vi "GPSDO53335ATester.vi"() -> ()   [LabVIEW 2015]
uses:
  <vilib>/Instr/_visa.llb/VISA Configure Serial Port (Instr).vi
panel:
  out "Measurement":cluster{"Measurment":ext, "Measurment":ext}(graph)
  out "Measurment":ext format="%.9e"
  in  "AC\nDC 2":bool
  in  "AC\nDC":bool
  in  "Gate Delay":ext=0.25 format="%.3f"
  out "CNT No Change Votes":dbl
  out "CNT Down Votes":dbl
  out "CNT Up Votes":dbl
  out "RS No Change Votes":dbl
  out "RS Down Votes":dbl
  out "Running Sum":dbl(graph)
  in  "Clear":bool
  in  "Baud Rate":dbl=115200.0
  in  "COM Port":refnum<visa-resource-name>
  out "Error Out":errorcluster
  in  "Error In":errorcluster
  out "Tracked Satellites":cluster{dbl, dbl}(graph)
  in  "Save DAC to EEPROM":bool
  in  "Reset GPS":bool
  in  "Set DAC":dbl
  in  "Update DAC":bool
  in  "Change Algorithim":bool
  out "UpTime":string
  out "Warmed Up?":bool
  out "Enforce Warmup":bool
  out "Algorithim In Use":string
  out "Antenna Status":string
  out "Time":string
  in  "Stop":bool
  out "Raw Data":string
  out "Date":string
  out "RS Up Votes":dbl
  out "Running Sum":dbl
  out "DAC Value":dbl
  out "Adjustments Made":dbl
  out "Samples":dbl
  out "Error (mHz)":dbl
  out "Count":cluster{dbl, dbl}(graph)
  out "Longitude":dbl format="%#_9g"
  out "Latitude":dbl
  out "Tracked Satellites":dbl
  out "Visible Satellites":dbl
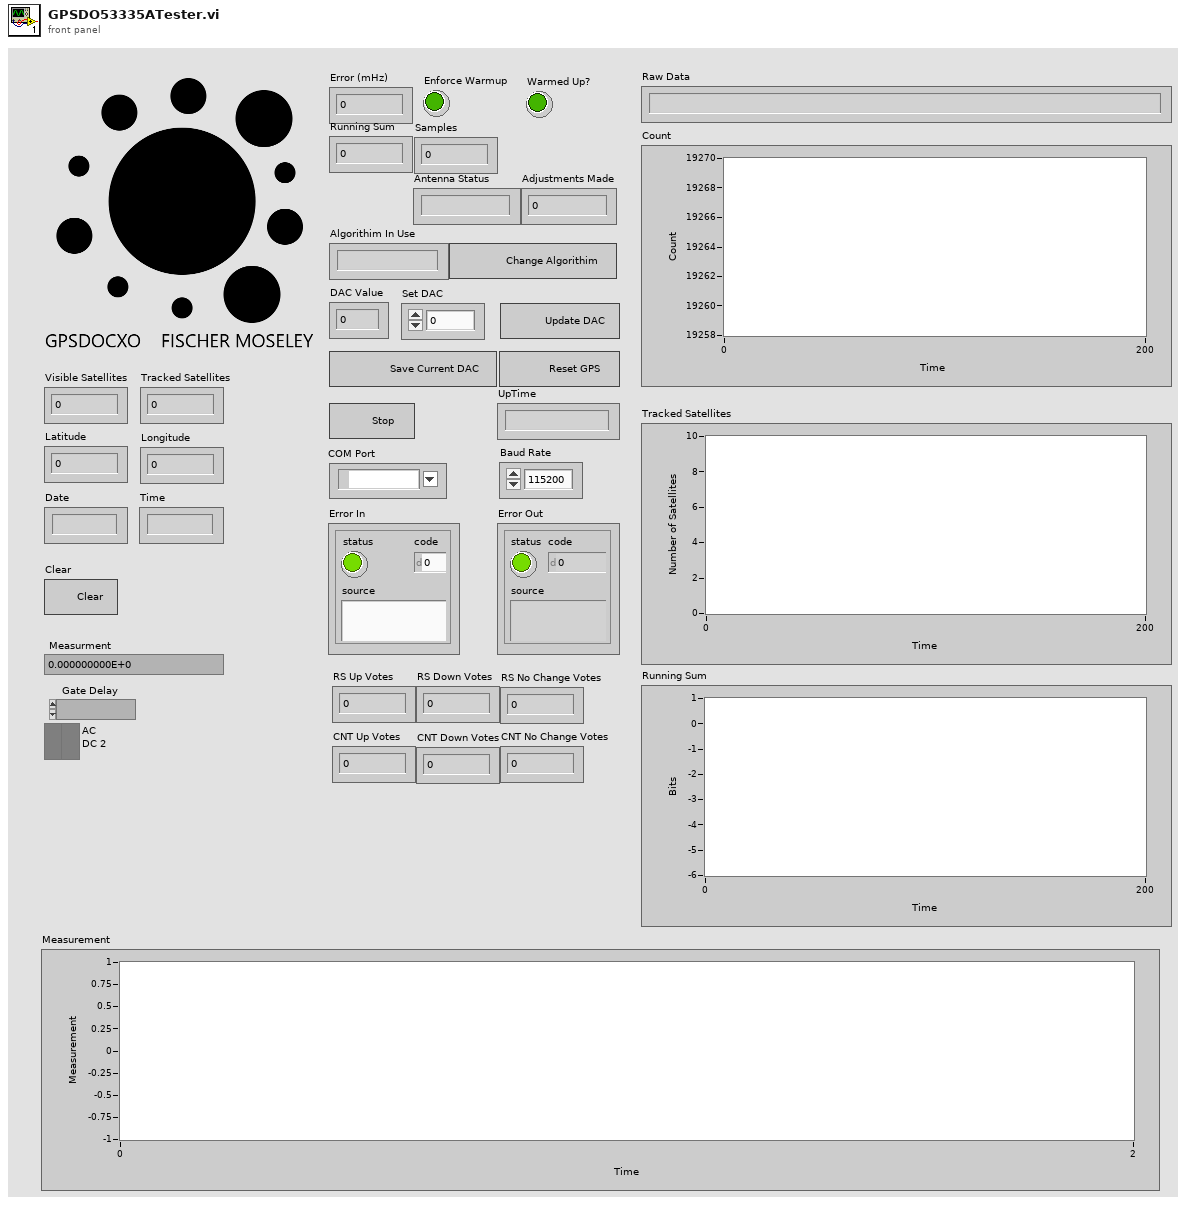
[diagram p1: front panel]
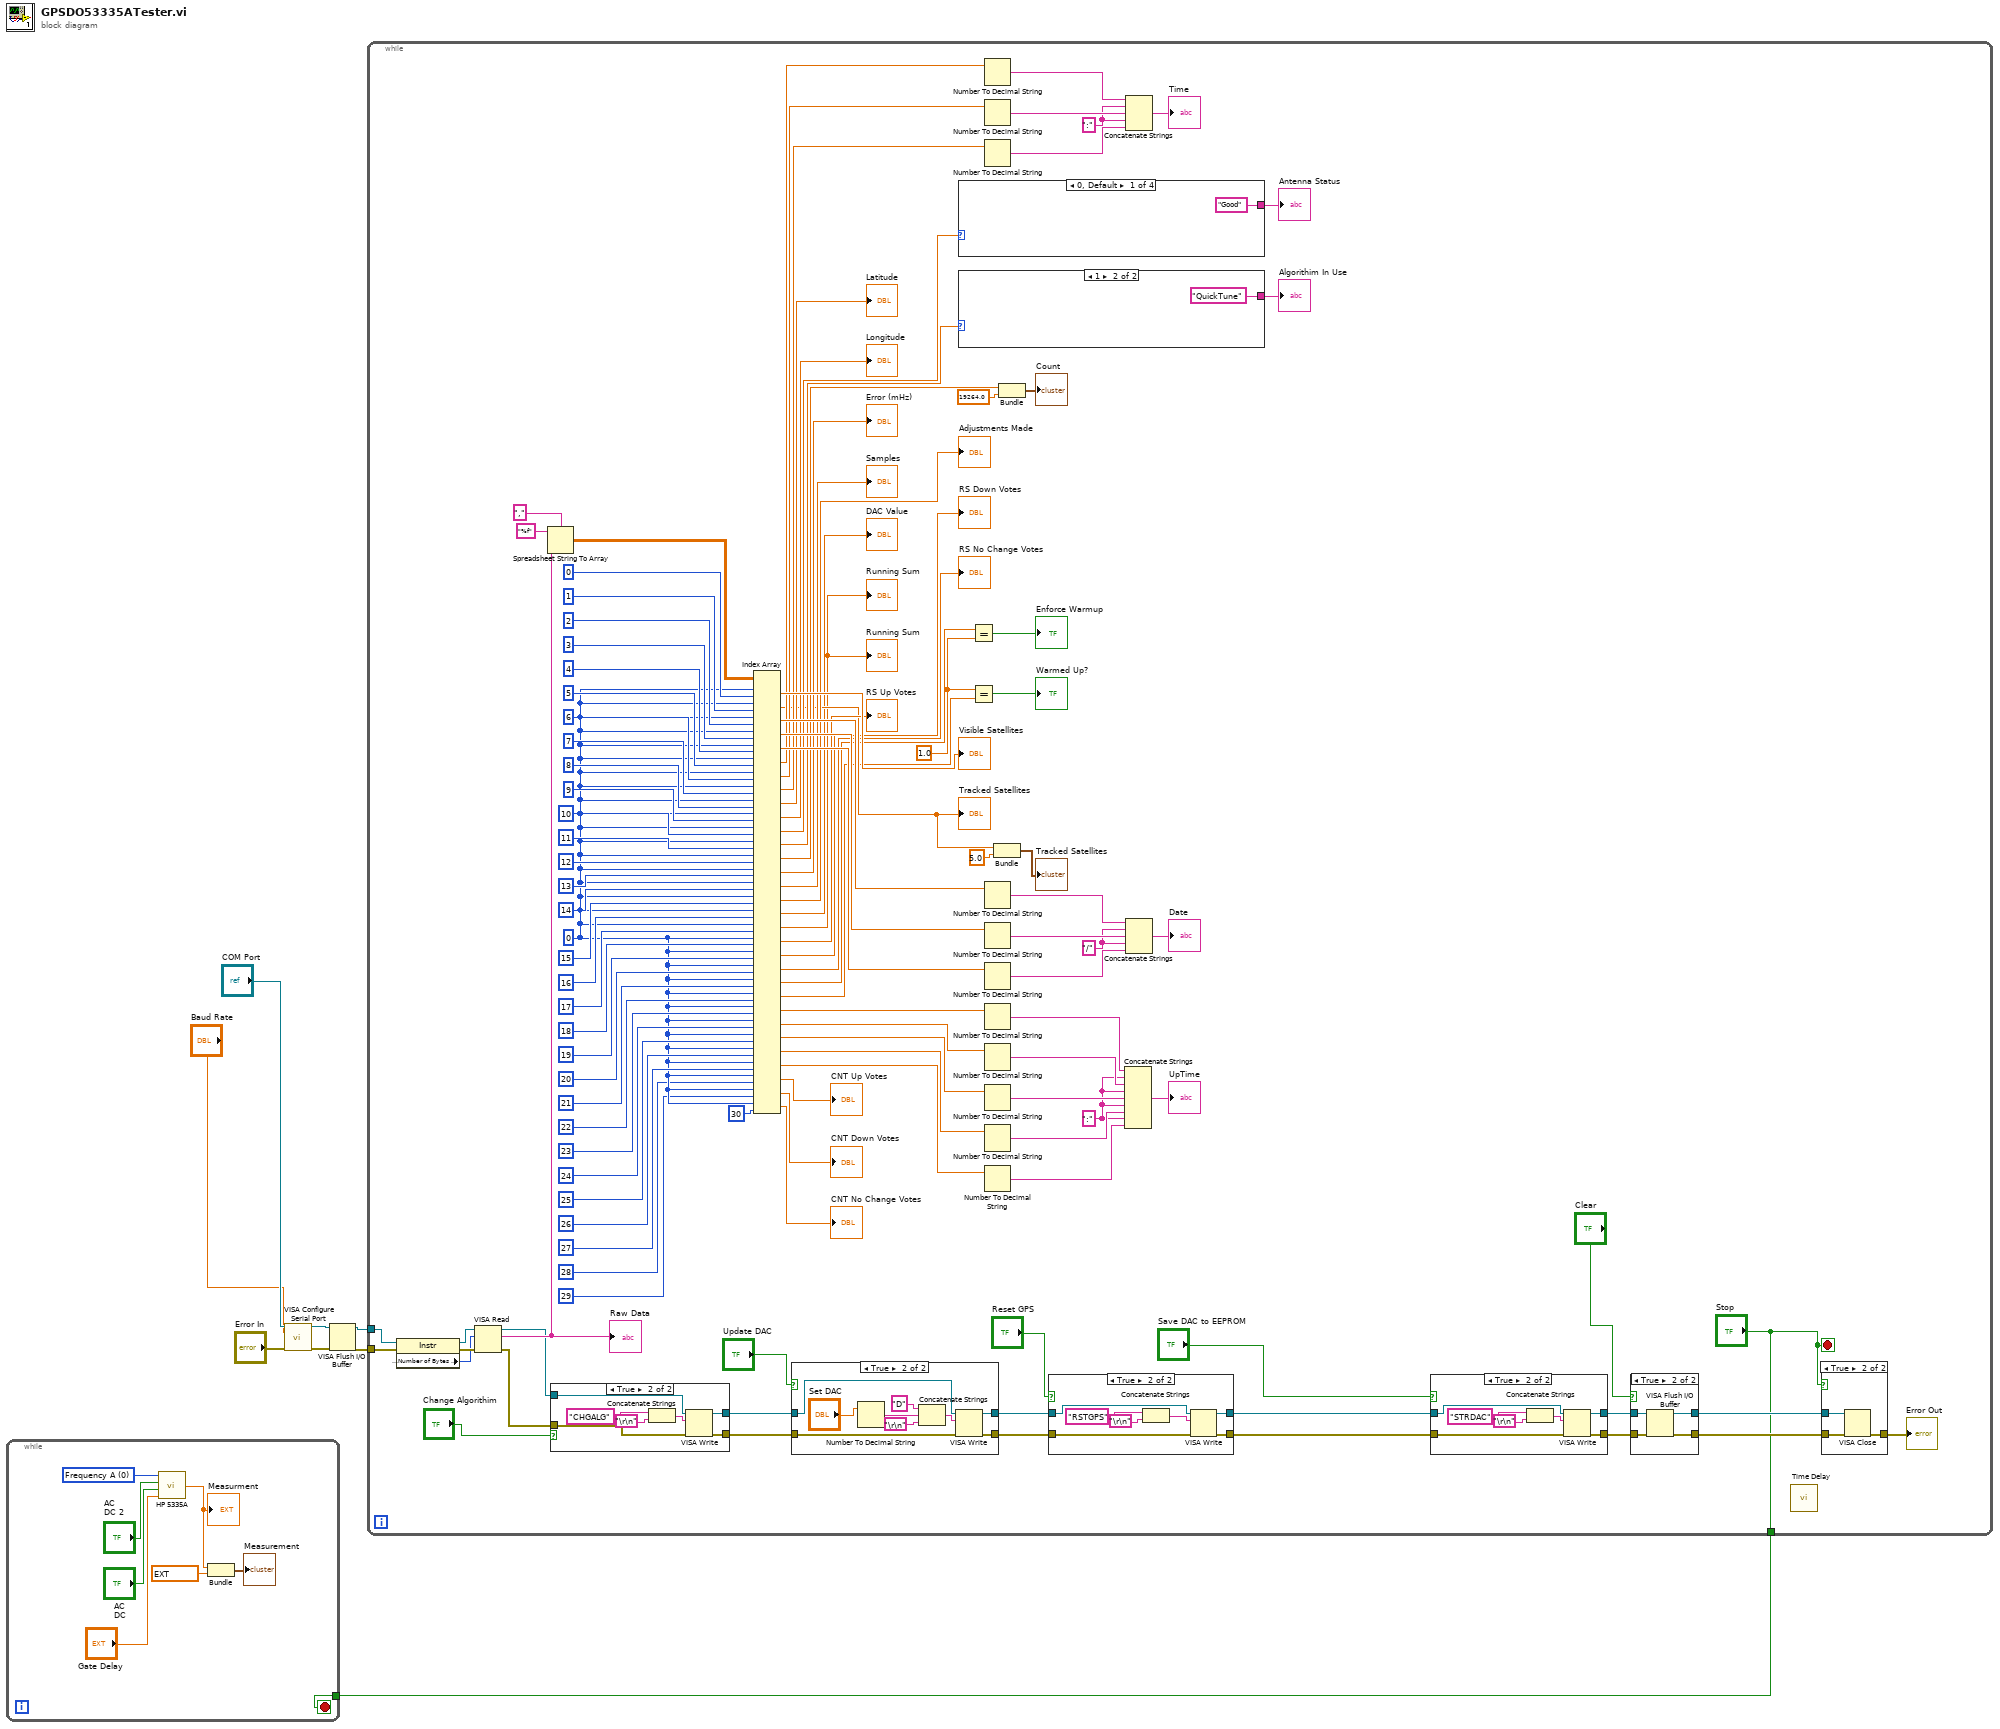
[diagram p0: block diagram]
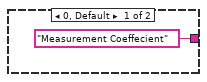
[diagram p7: hidden frame]
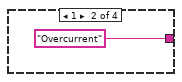
[diagram p8: hidden frame]
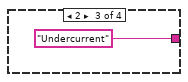
[diagram p9: hidden frame]
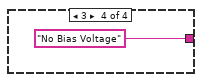
[diagram p10: hidden frame]
diagram:
  n1 = call-poly "VISA Configure Serial Port"("VISA resource name"="COM Port", "baud rate (9600)"="Baud Rate", "error in (no error)"="Error In") -> ("VISA resource name out"=w7:refnum<visa-resource-name>, "error out"=w8:errorcluster)  [unwired: 11 in]
  n2 = VISA Flush I/O Buffer(VISA resource name=w7, error in (no error)=w8) -> (VISA resource name out=w5:refnum<visa-resource-name>, error out=w6:errorcluster)  [unwired: 1 in]
  n3 = while {
    tunnel: w6 -> [w120]
    tunnel: w5 -> [w119]
    tunnel: ["Stop"] -> w1
    stop <- "Stop" stop-if-true
    w64 = ":" ("string")
    w73 = "/" ("string")
    w16 = 0 ("index (row)")
    w107 = ":" ("string")
    w114 = 1.0 ("y")
    n4 = property class="Instr"(reference=w119, error in=w120) -> (reference out=w121:refnum<visa-resource-name>, error out=w123:errorcluster, "Serial Settings:Number of Bytes at Serial Port"=w122:u32)
    n5 = VISA Read(VISA resource name=w121, byte count=w122, error in (no error)=w123) -> (VISA resource name out=w51:refnum<visa-resource-name>, read buffer=w106:string, error out=w52:errorcluster)  [unwired: 1 out]
    "Raw Data" <- w106
    n6 = Spreadsheet String To Array(delimiter (Tab)=",", format string="%f", spreadsheet string=w106) -> (array=w62:dbl[][])  [unwired: 1 in]
    n7 = case shown="True" "Change Algorithim" {
      tunnel: [w162 w169] -> w50
      tunnel: [w161 w168] -> w49
      tunnel: w52 -> [w161 w167]
      tunnel: w51 -> [w162 w166]
      frame False {
      }
      frame True {
        n8 = Concatenate Strings("CHGALG" ("write buffer"), "\r\n") -> (w164:string)
        n9 = VISA Write(VISA resource name=w166, write buffer=w164, error in (no error)=w167) -> (VISA resource name out=w169:refnum<visa-resource-name>, error out=w168:errorcluster)  [unwired: 1 out]
      }
    }
    n10 = Index Array(array=w62, index (row) #1=w16, index (col) #1=0 ("disabled index (col)"), index (row) #2=w16, index (col) #2=1 ("disabled index (col)"), index (row) #3=w16, index (col) #3=2 ("disabled index (col)"), index (row) #4=w16, index (col) #4=3 ("disabled index (col)"), index (row) #5=w16, index (col) #5=4 ("disabled index (col)"), index (row) #6=w16, index (col) #6=5 ("disabled index (col)"), index (row) #7=w16, index (col) #7=6 ("disabled index (col)"), index (row) #8=w16, index (col) #8=7 ("disabled index (col)"), index (row) #9=w16, index (col) #9=8 ("index (col)"), index (row) #10=w16, index (col) #10=9 ("index (col)"), index (row) #11=w16, index (col) #11=10 ("index (col)"), index (row) #12=w16, index (col) #12=11 ("index (col)"), index (row) #13=w16, index (col) #13=12 ("index (col)"), index (row) #14=w16, index (col) #14=13 ("index (col)"), index (row) #15=w16, index (col) #15=14 ("index (col)"), index (row) #16=w16, index (col) #16=15 ("index (col)"), index (row) #17=w16, index (col) #17=16 ("index (col)"), index (row) #18=w16, index (col) #18=17 ("index (col)"), index (row) #19=w16, index (col) #19=18 ("index (col)"), index (row) #20=w16, index (col) #20=19 ("index (col)"), index (row) #21=w16, index (col) #21=20 ("index (col)"), index (row) #22=w16, index (col) #22=21 ("index (col)"), index (row) #23=w16, index (col) #23=22 ("index (col)"), index (row) #24=w16, index (col) #24=23 ("index (col)"), index (row) #25=w16, index (col) #25=24 ("index (col)"), index (row) #26=w16, index (col) #26=25 ("index (col)"), index (row) #27=w16, index (col) #27=26 ("disabled index (col)"), index (row) #28=w16, index (col) #28=27 ("disabled index (col)"), index (row) #29=w16, index (col) #29=28 ("disabled index (col)"), index (row) #30=w16, index (col) #30=29 ("disabled index (col)"), index (row) #31=w16, index (col) #31=30 ("disabled index (col)")) -> (element #1=→"Visible Satellites":dbl, element #2=w37:dbl, element #3=w78:dbl, element #4=w76:dbl, element #5=w71:dbl, element #6=w70:dbl, element #7=w69:dbl, element #8=w68:dbl, element #9=→"Latitude":dbl, element #10=→"Longitude":dbl, element #11=w59:dbl, element #12=w58:dbl, element #13=w40:dbl, element #14=→"Error (mHz)":dbl, element #15=→"Samples":dbl, element #16=→"Adjustments Made":dbl, element #17=→"DAC Value":dbl, element #18=→"Running Sum" →"Running Sum":dbl, element #19=→"RS Up Votes":dbl, element #20=→"RS Down Votes":dbl, element #21=→"RS No Change Votes":dbl, element #22=w24:dbl, element #23=w23:dbl, element #24=w22:dbl, element #25=w21:dbl, element #26=w20:dbl, element #27=w19:dbl, element #28=w18:dbl, element #29=→"CNT Up Votes":dbl, element #30=→"CNT Down Votes":dbl, element #31=→"CNT No Change Votes":dbl)
    "Tracked Satellites" <- w37
    n11 = case shown="True" "Update DAC" {
      tunnel: [w151 w160] -> w47
      tunnel: [w150 w159] -> w46
      tunnel: w49 -> [w150 w158]
      tunnel: w50 -> [w151 w157]
      frame False {
      }
      frame True {
        n12 = Number To Decimal String(number="Set DAC") -> (decimal integer string=w152:string)  [unwired: 1 in]
        n13 = Concatenate Strings("D" ("write buffer"), w152, "\r\n") -> (w155:string)
        n14 = VISA Write(VISA resource name=w157, write buffer=w155, error in (no error)=w158) -> (VISA resource name out=w160:refnum<visa-resource-name>, error out=w159:errorcluster)  [unwired: 1 out]
      }
    }
    n15 = case shown="0, Default" w59 {
      tunnel: ["Good" ("Antenna Status") "Overcurrent" ("Antenna Status") "Undercurrent" ("Antenna Status") "No Bias Voltage" ("Antenna Status")] -> w118
      frame 0, Default {
      }
      frame 1 {
      }
      frame 2 {
      }
      frame 3 {
      }
    }
    "Antenna Status" <- w118
    n16 = case shown="1" w58 {
      tunnel: ["Measurement Coeffecient" ("Algorithim In Use") "QuickTune" ("Algorithim In Use")] -> w117
      frame 0, Default {
      }
      frame 1 {
      }
    }
    "Algorithim In Use" <- w117
    n17 = Equal?(x=w24, y=w114) -> (x = y?=→"Enforce Warmup":bool)
    n18 = Equal?(x=w114, y=w23) -> (x = y?=→"Warmed Up?":bool)
    n19 = Number To Decimal String(number=w70) -> (decimal integer string=w67:string)  [unwired: 1 in]
    n20 = Number To Decimal String(number=w69) -> (decimal integer string=w66:string)  [unwired: 1 in]
    n21 = Number To Decimal String(number=w68) -> (decimal integer string=w65:string)  [unwired: 1 in]
    n22 = Number To Decimal String(number=w78) -> (decimal integer string=w77:string)  [unwired: 1 in]
    n23 = Number To Decimal String(number=w76) -> (decimal integer string=w75:string)  [unwired: 1 in]
    n24 = Number To Decimal String(number=w71) -> (decimal integer string=w74:string)  [unwired: 1 in]
    n25 = Number To Decimal String(number=w22) -> (decimal integer string=w113:string)  [unwired: 1 in]
    n26 = Number To Decimal String(number=w21) -> (decimal integer string=w112:string)  [unwired: 1 in]
    n27 = Number To Decimal String(number=w20) -> (decimal integer string=w111:string)  [unwired: 1 in]
    n28 = Number To Decimal String(number=w19) -> (decimal integer string=w110:string)  [unwired: 1 in]
    n29 = Number To Decimal String(number=w18) -> (decimal integer string=w109:string)  [unwired: 1 in]
    n30 = Bundle(w37, "element"=5.0) -> (→"Tracked Satellites":cluster{dbl, "element":dbl})  [unwired: 1 in]
    n31 = Bundle(w40, "element"=19264.0) -> (→"Count":cluster{dbl, "element":dbl})  [unwired: 1 in]
    n32 = case shown="True" "Reset GPS" {
      tunnel: [w142 w149] -> w44
      tunnel: [w141 w148] -> w43
      tunnel: w46 -> [w141 w147]
      tunnel: w47 -> [w142 w146]
      frame False {
      }
      frame True {
        n33 = Concatenate Strings("RSTGPS" ("write buffer"), "\r\n") -> (w144:string)
        n34 = VISA Write(VISA resource name=w146, write buffer=w144, error in (no error)=w147) -> (VISA resource name out=w149:refnum<visa-resource-name>, error out=w148:errorcluster)  [unwired: 1 out]
      }
    }
    n35 = Concatenate Strings(w113, w107, w112, w107, w111, w107, w110, w107, w109) -> (→"UpTime":string)
    n36 = Concatenate Strings(w67, w64, w66, w64, w65) -> (→"Time":string)
    n37 = Concatenate Strings(w77, w73, w75, w73, w74) -> (→"Date":string)
    n38 = case shown="True" "Save DAC to EEPROM" {
      tunnel: [w133 w140] -> w34
      tunnel: [w132 w139] -> w33
      tunnel: w43 -> [w132 w138]
      tunnel: w44 -> [w133 w137]
      frame False {
      }
      frame True {
        n39 = Concatenate Strings("STRDAC" ("write buffer"), "\r\n") -> (w135:string)
        n40 = VISA Write(VISA resource name=w137, write buffer=w135, error in (no error)=w138) -> (VISA resource name out=w140:refnum<visa-resource-name>, error out=w139:errorcluster)  [unwired: 1 out]
      }
    }
    n41 = case shown="True" "Clear" {
      tunnel: [w127 w129] -> w32
      tunnel: [w126 w128] -> w31
      tunnel: w33 -> [w126 w131]
      tunnel: w34 -> [w127 w130]
      frame False {
      }
      frame True {
        n42 = VISA Flush I/O Buffer(VISA resource name=w130, error in (no error)=w131) -> (VISA resource name out=w129:refnum<visa-resource-name>, error out=w128:errorcluster)  [unwired: 1 in]
      }
    }
    n43 = call "Time Delay"() -> ()  [unwired: 11 in, 1 out]
    n44 = case shown="True" "Stop" {
      tunnel: w32 -> [_ w179]
      tunnel: w31 -> [w176 w177]
      tunnel: [w176 w178] -> w35
      frame False {
      }
      frame True {
        n45 = VISA Close(VISA resource name=w179, error in (no error)=w177) -> (error out=w178:errorcluster)
      }
    }
    "Error Out" <- w35
  }
  n46 = while {
    tunnel: w1 -> [w180]
    stop <- w180 stop-if-true
    w187 = i16 0 items=["Frequency A", "Frequency C", "Period A", "Time A to B", "1/(Time A to B)", "Ratio A/B", "Ratio C/A", "Pulse Width A", "Rise/Fall A", "Duty Cycle A"] ("function (freqA:0)")
    n47 = call <instrlib>:"HP 5335A.vi"("Gate Delay"="Gate Delay", 2:"AC\nDC"="AC\nDC", 3:"AC\nDC"="AC\nDC 2", "function (freqA:0)"=w187) -> ("Measurment"=w183:ext)
    "Measurment" <- w183
    n48 = Bundle("Measurment"=w183, "Measurment"=ext 10000000.0) -> (→"Measurement":cluster{"Measurment":ext, "Measurment":ext})  [unwired: 1 in]
  }
